vi "WPI_MotorControlGetSetRefNum.vi"(8 "error in (no error)":errorcluster, 9 "menu":T1=enum."get", 10 "refnum name":string, 11 "MotorControlDeviceRef":T2={"DeviceStatus"={"status"=FALSE, "code"=0, "source"=""}, "Type"=enum."PWM", "PWM"={"PWM Channel"=enum."PWM 1", "DeadBand"={"Name"="", "maxPositivePwm"=0, "minPositivePwm"=0, "centerPwm"=0, "maxNegativePwm"=0, "minNegativePwm"=0, "angularRange"=0}}, "CAN"={"Device Number"=0, "SetOutput VI Ref"=variant(enum8{"Percent VBus", "Current", "Speed", "Position", "Voltage"} enum."Percent VBus"), "GetOutput VI Ref"=variant(refnum<k1> refnum), "Enable VI Ref"=variant(dbl 12.0), "Disable VI Ref"=variant(enum8{"Percent VBus", "Speed", "Position", "Slave", "Unchanged / Invalid", "Voltage Compensation", "Current", "Motion Profile"} enum."Percent VBus"), "Data"=variant}, "Invert"=FALSE, "DIO PWM"={"PWM \"Enable\" Channel"=enum."Invalid", "DIOChannel"=enum."Invalid", "PWM Rate"=0.0}}) -> (0 "error out":errorcluster, 2 "refnum names":string[](array[string]), 3 "MotorControlDeviceRef":T2={"DeviceStatus"={"status"=FALSE, "code"=0, "source"=""}, "Type"=enum."PWM", "PWM"={"PWM Channel"=enum."PWM 1", "DeadBand"={"Name"="", "maxPositivePwm"=0, "minPositivePwm"=0, "centerPwm"=0, "maxNegativePwm"=0, "minNegativePwm"=0, "angularRange"=0}}, "CAN"={"Device Number"=0, "SetOutput VI Ref"=variant(enum8{"Percent VBus", "Current", "Speed", "Position", "Voltage"} enum."Percent VBus"), "GetOutput VI Ref"=variant(refnum<k1> refnum), "Enable VI Ref"=variant(dbl 12.0), "Disable VI Ref"=variant(enum8{"Percent VBus", "Speed", "Position", "Slave", "Unchanged / Invalid", "Voltage Compensation", "Current", "Motion Profile"} enum."Percent VBus"), "Data"=variant}, "Invert"=FALSE, "DIO PWM"={"PWM \"Enable\" Channel"=enum."Invalid", "DIOChannel"=enum."Invalid", "PWM Rate"=0.0}})   [LabVIEW 2017]
doc: "Sets a reference into a registry, gets a reference from a registry, or deletes a reference from a registry. The reference is accessed by name, and can be given any unique name.\n\nThis software is licensed. Open the labview\\readme\\WPI Robotics Library Open Source License.txt file for more information."
uses:
  <vilib>/Rock Robotics/WPI/MotorControl/WPI_MotorControlDeviceRef.ctl
  <vilib>/Rock Robotics/WPI/MotorControl/WPI_MotorControlType.ctl
  <vilib>/Rock Robotics/SystemInterfaces/DIO/FPGA_DIOPWMChannel.ctl
  <vilib>/Rock Robotics/WPI/PWM/WPI_PWMDeadband.ctl
  <vilib>/Rock Robotics/SystemInterfaces/DIO/FPGA_DIOChannel.ctl
  <vilib>/Rock Robotics/WPI/Utilities/Refnum Registry Operation.ctl
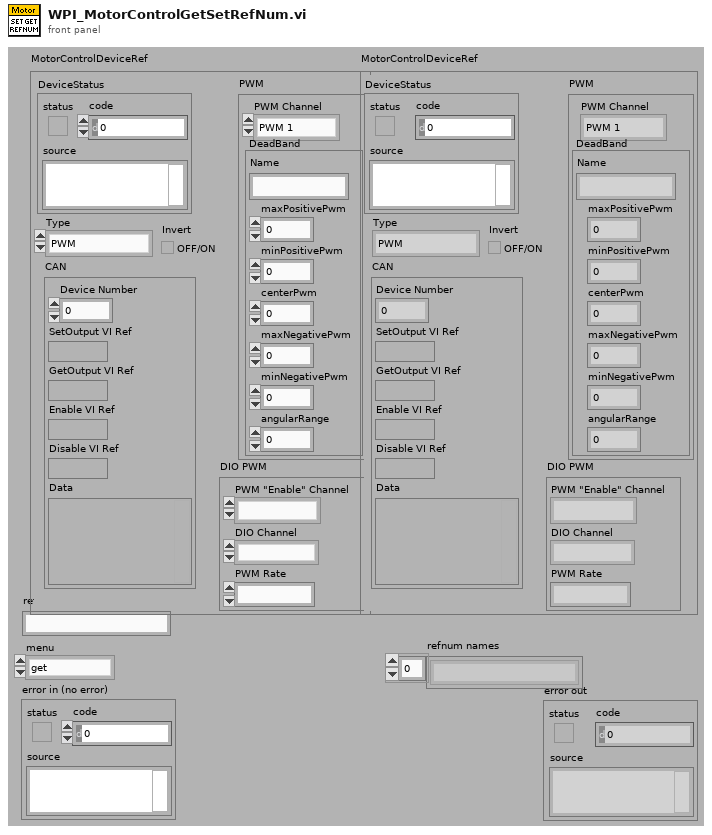
[diagram p1: front panel]
types:
  T1 = typedef "Refnum Registry Operation.ctl" = enum16{"set", "get", "delete", "get all names", "read name"}
  T2 = typedef "WPI_MotorControlDeviceRef.ctl" = cluster{"DeviceStatus":errorcluster, "Type":T3, "PWM":cluster{"PWM Channel":T4, "DeadBand":T5}, "CAN":cluster{"Device Number":u8, "SetOutput VI Ref":variant, "GetOutput VI Ref":variant, "Enable VI Ref":variant, "Disable VI Ref":variant, "Data":variant}, "Invert":bool, "DIO PWM":cluster{"PWM \"Enable\" Channel":T4, "DIOChannel":T6, "PWM Rate":dbl}}
  T3 = typedef "WPI_MotorControlType.ctl" = enum16{"PWM", "CAN", "DIO PWM"}
  T4 = typedef "FPGA_DIOPWMChannel.ctl" = enum8{"PWM 0", "PWM 1", "PWM 2", "PWM 3", "PWM 4", "PWM 5", "PWM 6", "PWM 7", "PWM 8", "PWM 9", "PWM MXP 0", "PWM MXP 1", "PWM MXP 2", "PWM MXP 3", "PWM MXP 4", "PWM MXP 5", "PWM MXP 6", "PWM MXP 7", "PWM MXP 8", "PWM MXP 9", "Invalid"}
  T5 = typedef "WPI_PWMDeadband.ctl" = cluster{"Name":string, "maxPositivePwm":i32, "minPositivePwm":i32, "centerPwm":i32, "maxNegativePwm":i32, "minNegativePwm":i32, "angularRange":u16}
  T6 = typedef "FPGA_DIOChannel.ctl" = enum8{"DIO 0", "DIO 1", "DIO 2", "DIO 3", "DIO 4", "DIO 5", "DIO 6", "DIO 7", "DIO 8", "DIO 9", "DIO MXP 0", "DIO MXP 1", "DIO MXP 2", "DIO MXP 3", "DIO MXP 4", "DIO MXP 5", "DIO MXP 6", "DIO MXP 7", "DIO MXP 8", "DIO MXP 9", "DIO MXP 10", "DIO MXP 11", "DIO MXP 12", "DIO MXP 13", "DIO MXP 14", "DIO MXP 15", "SPI Port CS1", "SPI Port CS2", "SPI Port CS3", "SPI Port MISO", "SPI Port MOSI", "Invalid"}
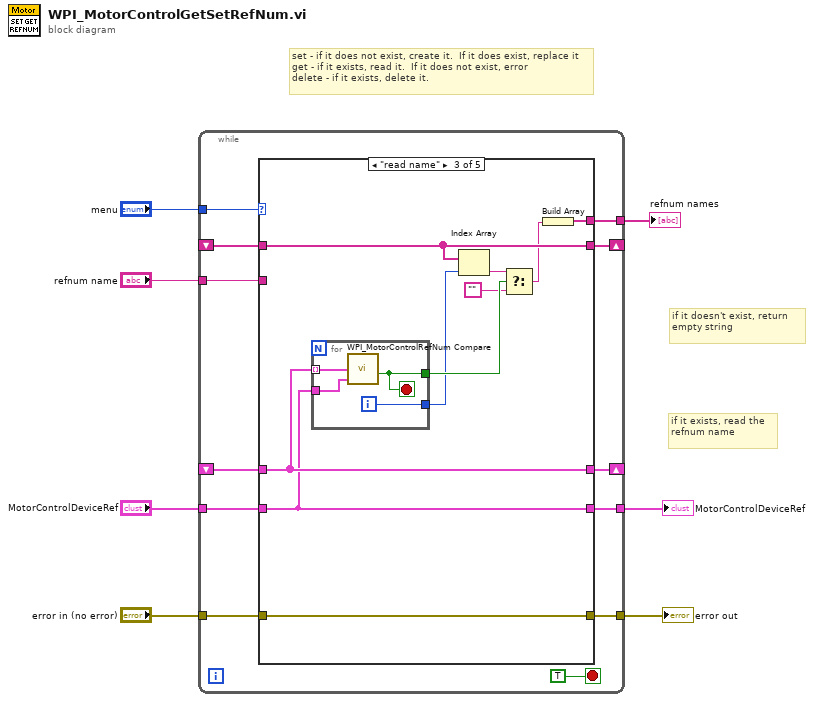
[diagram p0: block diagram]
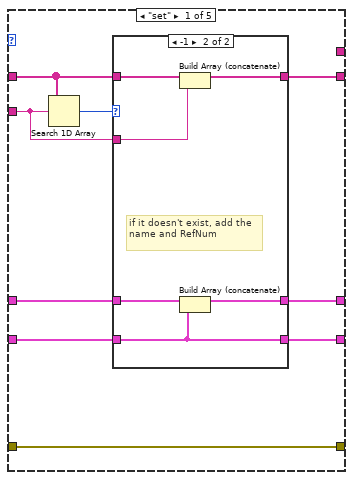
[diagram p2: hidden frame]
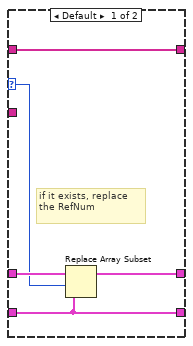
[diagram p3: hidden frame]
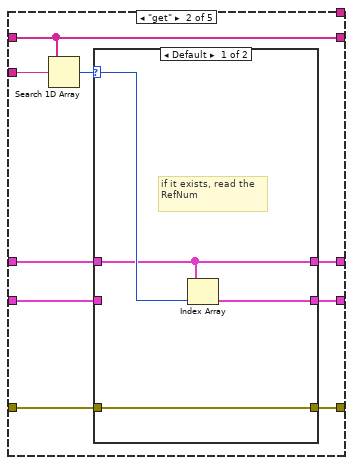
[diagram p4: hidden frame]
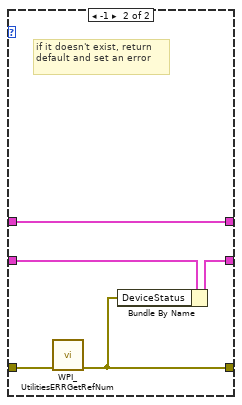
[diagram p5: hidden frame]
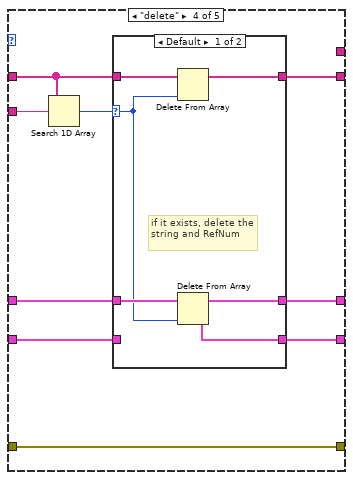
[diagram p6: hidden frame]
diagram:
  # "if it exists, read the refnum name"
  # "if it doesn't exist, return empty string"
  # "set - if it does not exist, create it.  If it does exist, replace it\nget - if it exists, read it.  If it does not exist, error\ndelete - if it exists, delete it."
  n1 = while {
    tunnel: "MotorControlDeviceRef" -> [w19]
    tunnel: "refnum name" -> [w12]
    tunnel: "error in (no error)" -> [w11]
    shift-right: [w18] -> _
    shift-left: _ -> [w17]
    tunnel: [w16] -> w5
    tunnel: "menu" -> [w15]
    shift-right: [w14] -> _
    shift-left: _ -> [w13]
    tunnel: [w10] -> w3
    tunnel: [w8] -> w1
    stop <- TRUE stop-if-true
    n2 = case shown="\"read name\"" w15 {
      tunnel: w19 -> [w23 w46 w65 w76 w92]
      tunnel: [w22 w45 w66 w75 w93] -> w18
      tunnel: w17 -> [w24 w47 w66 w77 w93]
      tunnel: [w21 w44 w65 w74 w92] -> w16
      tunnel: [w28 w43 w64 w80 w90] -> w14
      tunnel: w13 -> [w27 w43 w64 w79 w90]
      tunnel: w12 -> [w25 w40 _ w72 _]
      tunnel: [w20 w41 w67 w73 w91] -> w10
      tunnel: w11 -> [w20 w42 w67 w73 w91]
      tunnel: [_ _ w59 _ w90] -> w8
      frame "set" {
        n3 = Search 1D Array(1D array=w27, element=w25) -> (index of element=w26:i32)  [unwired: 1 out]
        n4 = case shown="-1" w26 {
          selector: w26 -> [w31 _]
          tunnel: [w33 w39] -> w28
          tunnel: w27 -> [w33 w38]
          tunnel: w25 -> [_ w34]
          tunnel: w24 -> [w32 w37]
          tunnel: w23 -> [w29 w35]
          tunnel: [w30 w36] -> w22
          tunnel: [w29 w35] -> w21
          frame Default {
            # "if it exists, replace the RefNum"
            n5 = Replace Array Subset(array=w32, new element=w29, index=w31) -> (w30:T2[])
          }
          frame -1 {
            # "if it doesn't exist, add the name and RefNum"
            n6 = Build Array (concatenate)(w38, w34) -> (w39:string[])
            n7 = Build Array (concatenate)(w37, w35) -> (w36:T2[])
          }
        }
      }
      frame "get" {
        n8 = Search 1D Array(1D array=w43, element=w40) -> (index of element=w48:i32)  [unwired: 1 out]
        n9 = case shown="Default" w48 {
          selector: w48 -> [w52 _]
          tunnel: w47 -> [w50 w57]
          tunnel: w46 -> [_ w55]
          tunnel: [w50 w57] -> w45
          tunnel: [w51 w54] -> w44
          tunnel: w42 -> [w49 w56]
          tunnel: [w49 w53] -> w41
          frame Default {
            # "if it exists, read the RefNum"
            n10 = Index Array(array=w50, index=w52) -> (element=w51:T2)
          }
          frame -1 {
            # "if it doesn't exist, return default and set an error"
            n11 = call <vilib>:"WPI_UtilitiesERRGetRefNum.vi"("error in (no error)"=w56) -> ("ERRGetRefNum"=w53:errorcluster)  [unwired: 10 out]
            n12 = Bundle By Name(cluster=w55, "DeviceStatus"=w53) -> (w54:T2)
          }
        }
      }
      frame "read name" {
        n13 = for {
          tunnel: w66 -> [w71] mode=indexing
          tunnel: w65 -> [w70]
          tunnel: [w68] -> w62
          tunnel: [w69] -> w60
          i -> [w69]
          stop <- w68 stop-if-true
          n14 = call <vilib>:"WPI_MotorControlRefNum Compare.vi"("MotorControlDeviceRef 1"=w71, "MotorControlDeviceRef 2"=w70) -> ("Equal?"=w68:bool)  [unwired: 4 out]
        }
        n15 = Index Array(array=w64, index=w60) -> (element=w63:string)
        n16 = Select(t=w63, s=w62, f="") -> (s? t:f=w58:string)
        n17 = Build Array(w58) -> (w59:string[])
      }
      frame "delete" {
        n18 = Search 1D Array(1D array=w79, element=w72) -> (index of element=w78:i32)  [unwired: 1 out]
        n19 = case shown="Default" w78 {
          selector: w78 -> [w81 _]
          tunnel: [w82 w88] -> w80
          tunnel: w79 -> [w83 w88]
          tunnel: w77 -> [w86 w87]
          tunnel: w76 -> [_ w89]
          tunnel: [w85 w87] -> w75
          tunnel: [w84 w89] -> w74
          frame Default {
            # "if it exists, delete the string and RefNum"
            n20 = Delete From Array(array=w83, index=w81) -> (array with subset deleted=w82:string[])  [unwired: 1 in, 1 out]
            n21 = Delete From Array(array=w86, index=w81) -> (deleted portion=w84:T2, array with subset deleted=w85:T2[])  [unwired: 1 in]
          }
          frame -1 {
            # "if it doesn't exist, do nothing"
          }
        }
      }
      frame "get all names" {
      }
    }
  }
  "error out" <- w3
  "MotorControlDeviceRef" <- w5
  "refnum names" <- w1
